vi "READ - File.vi"(0 "reference in":refnum<class "TDMS.lvclass">, 5 "error in (no error)":errorcluster, 7 "TDMS Path - READ":path) -> (13 "File Loaded":path, 14 "reference out":refnum<class "TDMS.lvclass">, 19 "error out":errorcluster)   [LabVIEW 2022 SP3, in "TDMS.lvclass"]
uses:
  TDMS.lvclass
  API/GSwFormDSP_class/functions/Attribute List.ctl
  API/GSwFormDSP_class/GSwFormDSP.lvclass
  API/Generic Utilities_class/Generic Utilities.lvclass
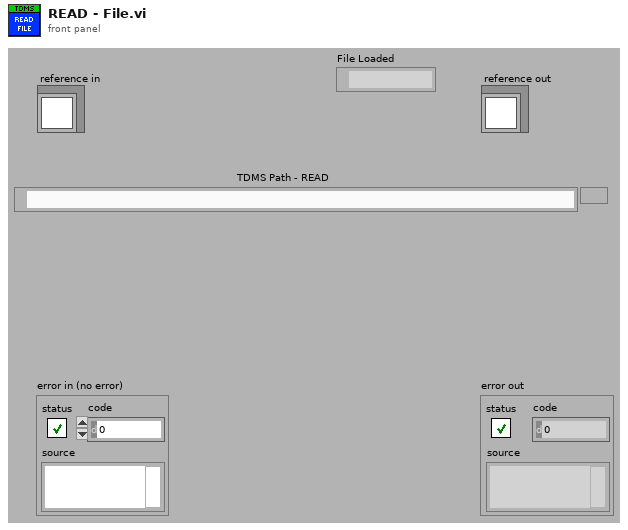
[diagram p1: front panel]
types:
  T1 = typedef "GSwFormDSP.lvclass/Attribute List.ctl" = string
  T2 = typedef "TDMS.lvclass/ObjectAttributesRef.ctl" = refnum<data-value>
  T3 = typedef "TDMS.lvclass/ObjectAttributes.ctl" = cluster{"Time Data":refnum<class "GSwFormDSP.lvclass">, "New Time Data Obj?":bool}
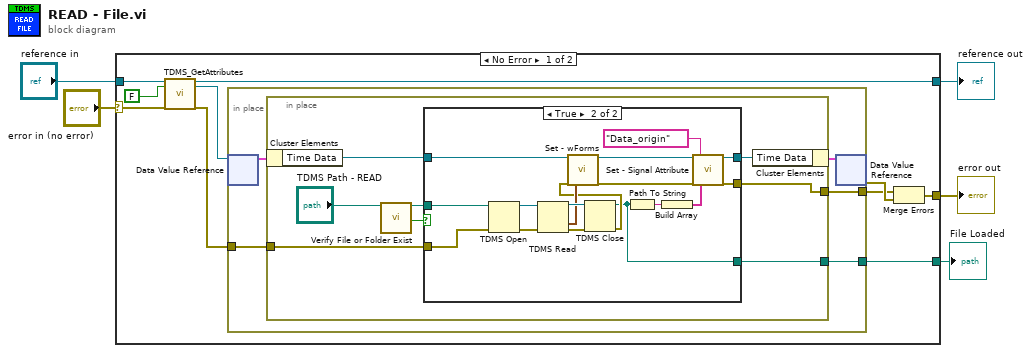
[diagram p0: block diagram]
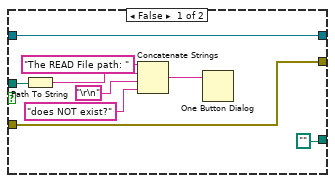
[diagram p2: hidden frame]
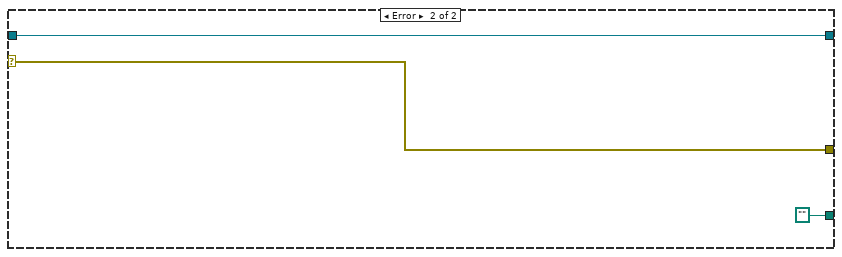
[diagram p3: hidden frame]
diagram:
  n1 = case shown="No Error" "error in (no error)" {
    selector: "error in (no error)" -> [w10 w57]
    tunnel: [w15 w57] -> w4
    tunnel: [w9 w56] -> w2
    tunnel: "reference in" -> [w12 w56]
    tunnel: [w6 path ""] -> w1
    frame No Error {
      n2 = call "TDMS_GetAttributes.vi"("reference in"=w12, "return data? (T)"=FALSE, "error in (no error)"=w10) -> ("reference out"=w9:refnum<class "TDMS.lvclass">, "attributes ref"=w8:T2, "error out"=w7:errorcluster)  [unwired: 13 in, 1 out]
      n3 = in-place {
        in-place-border: [w17] -> w13
        in-place-border: w7 -> [w18]
        in-place-border: [w16] -> w6
        n4 = in-place-dvr #1(w8) -> (w19:T3)  [unwired: 1 out]
        n5 = in-place {
          in-place-border: w18 -> [w23]
          in-place-border: [w22] -> w17
          in-place-border: [w21] -> w16
          n6 = in-place-cluster #2(w19) -> ("Time Data"=w24:refnum<class "GSwFormDSP.lvclass">)
          n7 = call "Verify File or Folder Exist.vi"("path"="TDMS Path - READ") -> ("dup path"=w28:path, "file or folder exists?"=w27:bool)  [unwired: 16 in, 1 out]
          n8 = case shown="True" w27 {
            tunnel: w24 -> [w37 w54]
            tunnel: [w37 w50] -> w25
            tunnel: w28 -> [w35 w43]
            tunnel: w23 -> [w36 w42]
            tunnel: [w36 w51] -> w22
            tunnel: [path "" w38] -> w21
            frame False {
              n9 = Path To String(path=w35) -> (string=w33:string)
              n10 = Concatenate Strings("The READ File path: ", w33, "\r\n", "does NOT exist?") -> (w30:string)
              n11 = One Button Dialog(message=w30) -> ()  [unwired: 1 in, 1 out]
            }
            frame True {
              n12 = TDMS Open(8:w42, 11:w43) -> (0:w49:errorcluster, 3:w48:refnum<k34>)  [unwired: 5 in]
              n13 = TDMS Read(0:w48, 11:w49) -> (4:w46:refnum<k34>, 10:w45:waveform(dbl)[], 15:w47:errorcluster)  [unwired: 6 in, 3 out]
              n14 = TDMS Close(8:w47, 11:w46) -> (0:w44:errorcluster, 3:w38:path)
              n15 = call "Set - wForms.vi"("reference in"=w54, "error in (no error)"=w44, "wForms"=w45) -> ("reference out"=w53:refnum<class "GSwFormDSP.lvclass">, "error out"=w52:errorcluster)  [unwired: 15 in]
              n16 = Path To String(path=w38) -> (string=w41:string)
              n17 = Build Array(w41) -> (w40:string[])
              n18 = call-dynamic "Set - Signal Attribute.vi"("reference in"=w53, "error in (no error)"=w52, "wForm Attributes"=T1 "Data_origin", "Attribute"=w40) -> ("reference in"=w50:refnum<class "GSwFormDSP.lvclass">, "error out"=w51:errorcluster)  [unwired: 14 in]
            }
          }
          n19 = in-place-cluster #2("Time Data"=w25) -> (w20:T3)
        }
        n20 = in-place-dvr #1(w20) -> (w14:errorcluster)  [unwired: 1 out]
      }
      n21 = Merge Errors(w13, w14) -> (w15:errorcluster)
    }
    frame Error {
    }
  }
  "error out" <- w4
  "reference out" <- w2
  "File Loaded" <- w1
